vi "Vecto Group Config.vi"(8 "error in (no error)":errorcluster, 11 "Group in":refnum<class "Group.lvclass">) -> (0 "error out":errorcluster, 2 "Vecto Group Config":refnum<class "Group Config.lvclass">, 3 "Group out":refnum<class "Group.lvclass">)   [LabVIEW 2020, in "VolatusConfig.lvlib" / "Group.lvclass"]
uses:
  Group.lvclass
  C:/dev/lv20CE/relink/lv-volatus/VolatusConfig/VolatusConfigElement/VolatusConfigElement.lvclass
  lv-vecto/Vecto/Group Config/Group Config.lvclass
  lv-vecto/Vecto/Group Info.ctl
  VolatusConfigElement/VolatusConfigElement.lvclass/VolatusConfigElement.ctl
  VolatusConfigElement/Element.vi
  VolatusConfigElement/Lookup Child by Name.vi
  Task/Task.lvclass
  Node/Node.lvclass
  Cluster/Cluster.lvclass
  System/System.lvclass
  Channel/Channel.lvclass
  lv-cdm/CDM-Config/Config Element/Lookup Child by Name.vi
  lv-cdm/CDM-Config/Config Element/Value (String).vi
  VolatusConfigElement/VolatusConfigElement.lvclass
  lv-vecto/VectoConfig/VectoConfig.lvlib
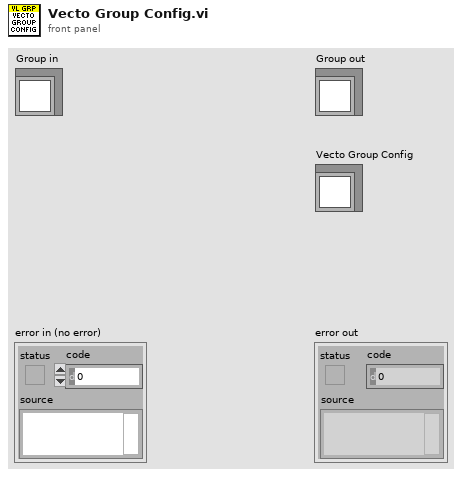
[diagram p1: front panel]
types:
  T1 = typedef "VectoConfig.lvlib/Group Info.ctl" = cluster{"System":string, "Cluster":string, "Node":string, "Task":string, "Name":string}
  T2 = typedef "VolatusConfig.lvlib/Group Type.ctl" = enum16{"Double", "String"}
  T3 = typedef "VolatusConfig.lvlib/Endpoint.ctl" = cluster{"Address":string, "Port":u16}
  T4 = cluster{"Name":string, "Resource":string, "Unit String":string}
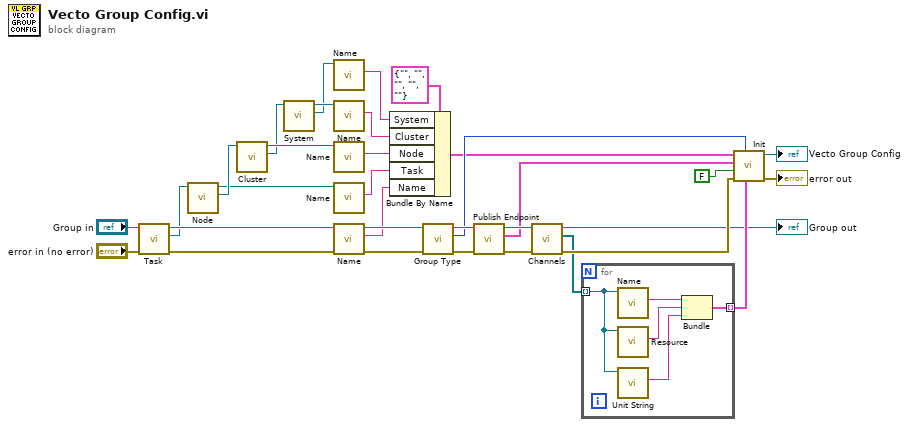
[diagram p0: block diagram]
diagram:
  n1 = call "Task.vi"("error in (no error)"="error in (no error)", "Group in"="Group in") -> ("error out"=w23:errorcluster, "Task"=w20:refnum<class "Task.lvclass">, "Group out"=w21:refnum<class "Group.lvclass">)  [unwired: 7 in]
  n2 = call "Node.vi"("Task in"=w20) -> ("Node"=w19:refnum<class "Node.lvclass">, "Task out"=w18:refnum<class "Task.lvclass">)  [unwired: 8 in, 1 out]
  n3 = call "Cluster.vi"("Node in"=w19) -> ("Cluster"=w16:refnum<class "Cluster.lvclass">, "Node out"=w17:refnum<class "Node.lvclass">)  [unwired: 8 in, 1 out]
  n4 = call "System.vi"("Cluster in"=w16) -> ("System"=w14:refnum<class "System.lvclass">, "Cluster out"=w15:refnum<class "Cluster.lvclass">)  [unwired: 8 in, 1 out]
  n5 = call "Name.vi"("VolatusConfigElement in"=w14) -> ("Name"=w6:string)  [unwired: 8 in, 2 out]
  n6 = call "Name.vi"("VolatusConfigElement in"=w15) -> ("Name"=w7:string)  [unwired: 8 in, 2 out]
  n7 = call "Name.vi"("VolatusConfigElement in"=w17) -> ("Name"=w10:string)  [unwired: 8 in, 2 out]
  n8 = call "Name.vi"("VolatusConfigElement in"=w18) -> ("Name"=w9:string)  [unwired: 8 in, 2 out]
  n9 = call "Name.vi"("error in (no error)"=w23, "VolatusConfigElement in"=w21) -> ("error out"=w29:errorcluster, "Name"=w8:string, "VolatusConfigElement out"=w32:refnum<class "Group.lvclass">)  [unwired: 7 in]
  n10 = Bundle By Name(cluster=T1 {"System"="", "Cluster"="", "Node"="", "Task"="", "Name"=""} ("Group Info"), "System"=w6, "Cluster"=w7, "Node"=w10, "Task"=w9, "Name"=w8) -> (w11:T1)
  n11 = call "Group Type.vi"("error in (no error)"=w29, "Group in"=w32) -> ("error out"=w28:errorcluster, "Group Type"=w24:T2, "Group out"=w31:refnum<class "Group.lvclass">)  [unwired: 7 in]
  n12 = call "Publish Endpoint.vi"("error in (no error)"=w28, "Group in"=w31) -> ("error out"=w27:errorcluster, "Publish Endpoint"=w12:T3, "Group out"=w30:refnum<class "Group.lvclass">)  [unwired: 7 in]
  n13 = call "Channels.vi"("error in (no error)"=w27, "Group in"=w30) -> ("error out"=w33:errorcluster, "Channels"=w26:refnum<class "Channel.lvclass">[], "Group out"=→"Group out":refnum<class "Group.lvclass">)  [unwired: 7 in]
  n14 = for {
    tunnel: w26 -> [w35] mode=indexing
    tunnel: [w36] -> w5 mode=indexing
    n15 = call "Name.vi"("VolatusConfigElement in"=w35) -> ("Name"=w38:string)  [unwired: 8 in, 2 out]
    n16 = call "Resource.vi"("Channel in"=w35) -> ("Resource"=w37:string)  [unwired: 8 in, 2 out]
    n17 = call "Unit String.vi"("Channel in"=w35) -> ("Unit String"=w34:string)  [unwired: 8 in, 2 out]
    n18 = Bundle("Name"=w38, "Resource"=w37, "Unit String"=w34) -> (w36:T4)  [unwired: 1 in]
  }
  n19 = call "Init.vi"("Channels"=w5, "Group Data Type"=w24, "error in (no error)"=w33, "Raw Values (T)"=FALSE, "Publish Config (None)"=w12, "Group Info"=w11) -> ("error out"=→"error out":errorcluster, "Group Config out"=→"Vecto Group Config":refnum<class "Group Config.lvclass">)  [unwired: 4 in]
